vi "Manager Camera Communication.vi"(8 "error in (no error)":errorcluster, 11 "Channel in":refnum<class "Channel.lvclass">) -> (0 "error out":errorcluster, 3 "Channel out":refnum<class "Channel.lvclass">)   [LabVIEW 2018, in "Channel.lvclass"]
doc: "Manage camera communication"
uses:
  Channel.lvclass
  Channel.lvclass/Channel.ctl
  State Machine/State Machine.lvclass/State Machine.ctl
  State Machine/State Machine.lvclass
  Simulated_CCD_Camera/Simulated Camera.lvclass
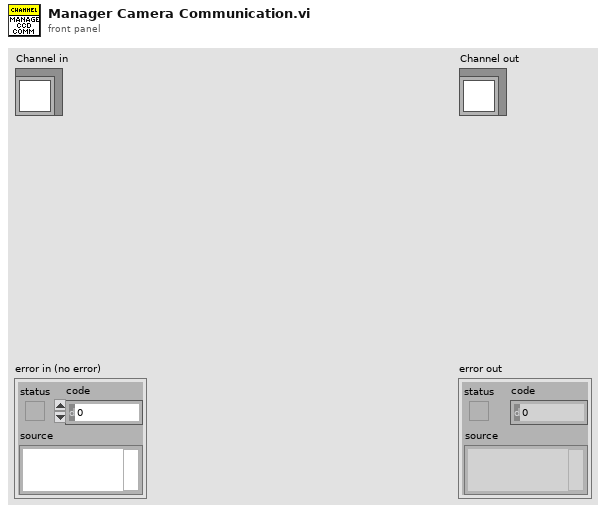
[diagram p1: front panel]
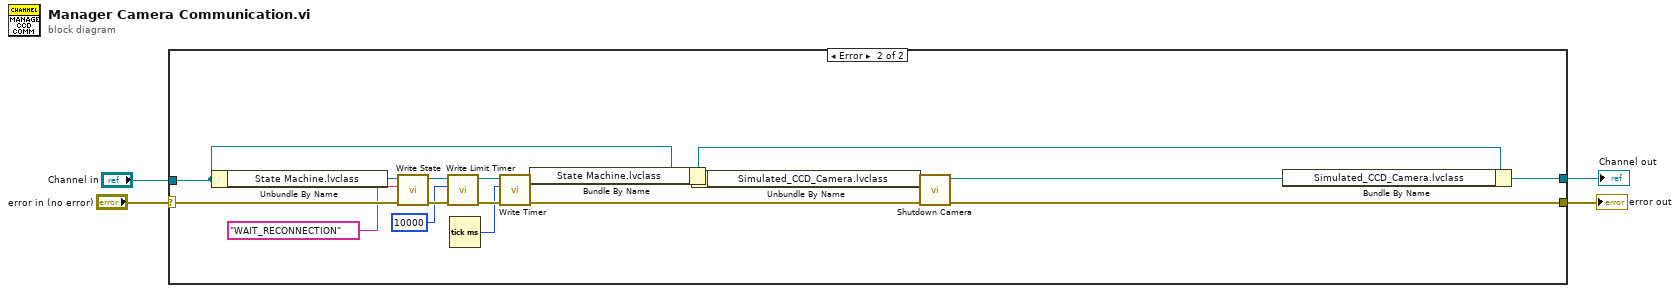
[diagram p0: block diagram]
diagram:
  n1 = case shown="Error" "error in (no error)" {
    selector: "error in (no error)" -> [w6 w21]
    tunnel: "Channel in" -> [w5 w22]
    tunnel: [w6 w7] -> w3
    tunnel: [w5 w23] -> w1
    frame No Error {
    }
    frame Error {
      n2 = Unbundle By Name(w22) -> ("State Machine.lvclass"=w20:refnum<class "State Machine.lvclass">)
      n3 = call-dynamic "Write State.vi"("error in (no error)"=w21, "State"="WAIT_RECONNECTION" ("CCD_STATUS"), "State Machine in"=w20) -> ("error out"=w16:errorcluster, "State Machine out"=w17:refnum<class "State Machine.lvclass">)  [unwired: 7 in]
      n4 = call "Write Limit Timer.vi"("error in (no error)"=w16, "Limit Timer"=u32 10000, "State Machine in"=w17) -> ("error out"=w13:errorcluster, "State Machine out"=w14:refnum<class "State Machine.lvclass">)  [unwired: 7 in]
      n5 = Tick Count (ms)() -> (millisecond timer value=w12:u32)
      n6 = call "Write Timer.vi"("error in (no error)"=w13, "Timer"=w12, "State Machine in"=w14) -> ("error out"=w11:errorcluster, "State Machine out"=w10:refnum<class "State Machine.lvclass">)  [unwired: 7 in]
      n7 = Bundle By Name(cluster=w22, "State Machine.lvclass"=w10) -> (w8:refnum<class "Channel.lvclass">)
      n8 = Unbundle By Name(w8) -> ("Simulated_CCD_Camera.lvclass"=w9:refnum<class "Simulated Camera.lvclass">)
      n9 = call-dynamic "Shutdown Camera.vi"("error in (no error)"=w11, "CCDCamera in"=w9) -> ("error out"=w7:errorcluster, "CCDCamera out"=w19:refnum<class "Simulated Camera.lvclass">)  [unwired: 8 in]
      n10 = Bundle By Name(cluster=w8, "Simulated_CCD_Camera.lvclass"=w19) -> (w23:refnum<class "Channel.lvclass">)
    }
  }
  "error out" <- w3
  "Channel out" <- w1
